vi "Get XML Path.vi"(11 "Project XML Editor in":refnum<class "Project XML Editor.lvclass">) -> (2 "XML Path":path, 3 "Project XML Editor out":refnum<class "Project XML Editor.lvclass">)   [LabVIEW 2019, in "LVLIBP CD XML Updater.lvlib" / "Project XML Editor.lvclass"]
uses:
  Project XML Editor.lvclass
  Project XML Editor.lvclass/Project XML Editor.ctl
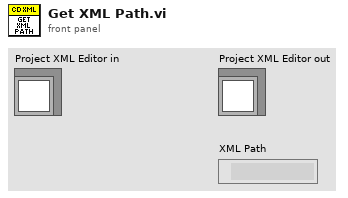
[diagram p1: front panel]
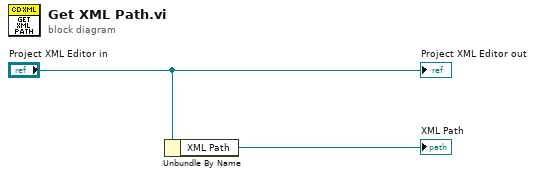
[diagram p0: block diagram]
diagram:
  n1 = Unbundle By Name("Project XML Editor in") -> ("XML Path"=→"XML Path":path)
  "Project XML Editor out" <- "Project XML Editor in"
